vi "Dequeue UI Loop.vi"(0 "Queue In":refnum<queue>, 5 "Test Results In":T1, 11 "error in (no error)":errorcluster) -> (6 "Test Results out":T1, 8 "Stop Button":bool, 15 "error out":errorcluster)   [LabVIEW 2016]
doc: "This VI handles the dequeueing of messages and message data from the producer/test loop."
uses:
  C:/Program Files (x86)/National Instruments/LabVIEW 2016/examples/Design Patterns/Queued Message Handler/support/QMH Fundamentals - Message Cluster.ctl
  controls/Test Results.ctl
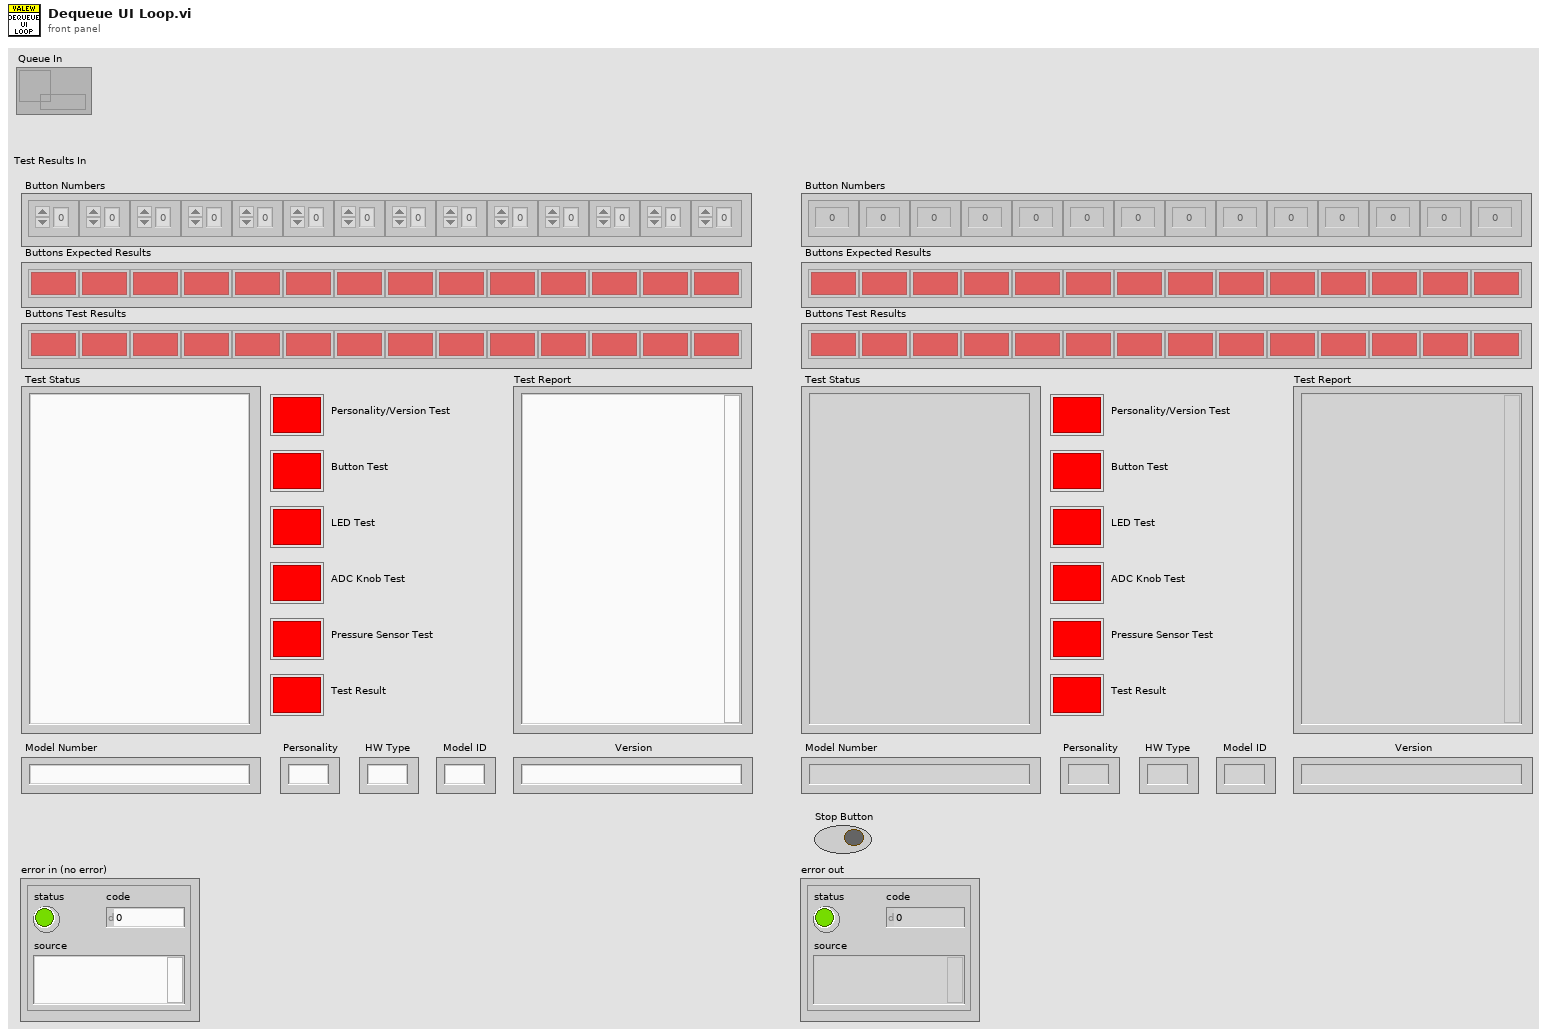
[diagram p1: front panel]
types:
  T1 = typedef "Test Results.ctl" = cluster{"Test Status":string, "Personality/Version Test ":bool, "Test Report":string, "Model Number":string, "Button Numbers":i32[], "Buttons Test Results":bool[], "Buttons Expected Results":bool[], "Model ID":string, "Personality":string, "HW Type":string, "Version":string, "Button Test":bool, "LED Test":bool, "ADC Knob Test":bool, "Pressure Sensor Test":bool, "Test Result":bool}
  T2 = typedef "QMH Fundamentals - Message Cluster.ctl" = cluster{"Message":string, "Message Data":variant}
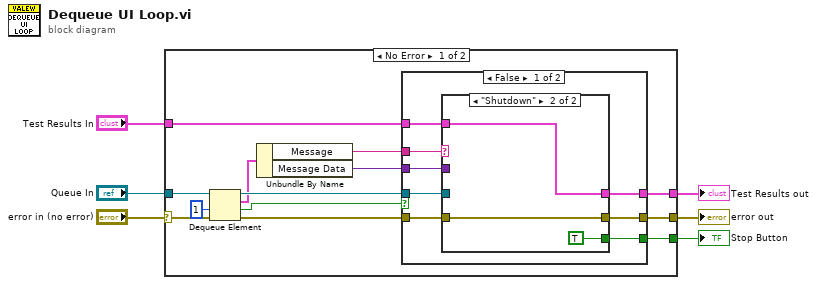
[diagram p0: block diagram]
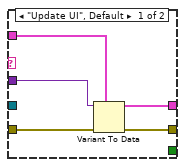
[diagram p2: hidden frame]
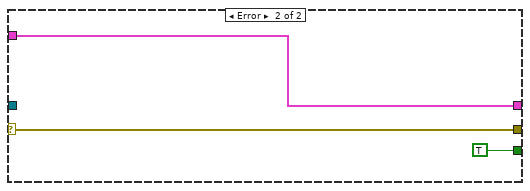
[diagram p4: hidden frame]
diagram:
  n1 = case shown="No Error" "error in (no error)" {
    selector: "error in (no error)" -> [w11 w40]
    tunnel: [w19 w40] -> w6
    tunnel: [w17 TRUE] -> w5
    tunnel: "Queue In" -> [w12 _]
    tunnel: "Test Results In" -> [w10 w38]
    tunnel: [w8 w38] -> w1
    frame No Error {
      n2 = Dequeue Element(queue=w12, timeout in ms (-1)=1, error in (no error)=w11) -> (queue out=w18:refnum<queue>, element=w13:T2, timed out?=w7:bool, error out=w16:errorcluster)
      n3 = Unbundle By Name(w13) -> ("Message"=w14:string, "Message Data"=w15:variant)
      n4 = case shown="False" w7 {
        tunnel: [w27 w37] -> w19
        tunnel: w18 -> [w26 _]
        tunnel: [w25 _] -> w17
        tunnel: w16 -> [w24 w37]
        tunnel: w15 -> [w23 _]
        tunnel: w14 -> [w22 _]
        tunnel: w10 -> [w21 w36]
        tunnel: [w20 w36] -> w8
        frame False {
          n5 = case shown="\"Shutdown\"" w22 {
            tunnel: w23 -> [w28 _]
            tunnel: w24 -> [w32 w33]
            tunnel: [_ TRUE] -> w25
            tunnel: w26 -> [_ _]
            tunnel: [w31 w33] -> w27
            tunnel: w21 -> [w30 w34]
            tunnel: [w29 w34] -> w20
            frame "Update UI", Default {
              n6 = Variant To Data(error in=w32, type=w30, Variant=w28) -> (data=w29:T1, error out=w31:errorcluster)
            }
            frame "Shutdown" {
            }
          }
        }
        frame True {
        }
      }
    }
    frame Error {
    }
  }
  "error out" <- w6
  "Stop Button" <- w5
  "Test Results out" <- w1
